vi "TopicRequest_Reply.vi"(2 "Subscriber":T1) -> (0 "XML":string)   [LabVIEW 2012]
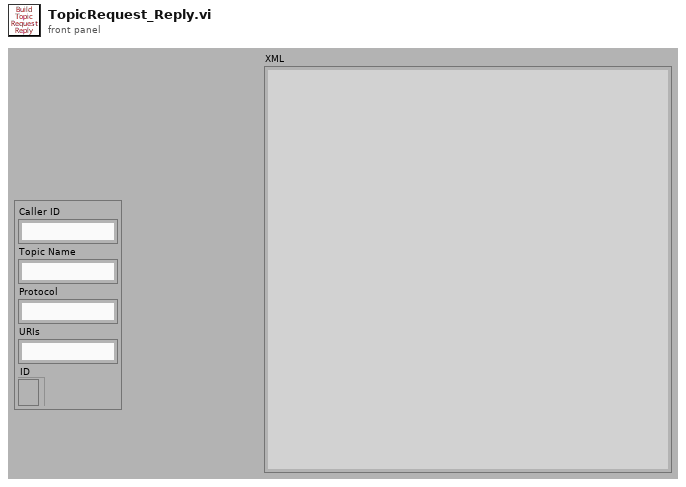
[diagram p1: front panel]
types:
  T1 = cluster{"Caller ID":string, "Topic Name":string, "Protocol":string, "URIs":string, "ID":refnum<k5>}
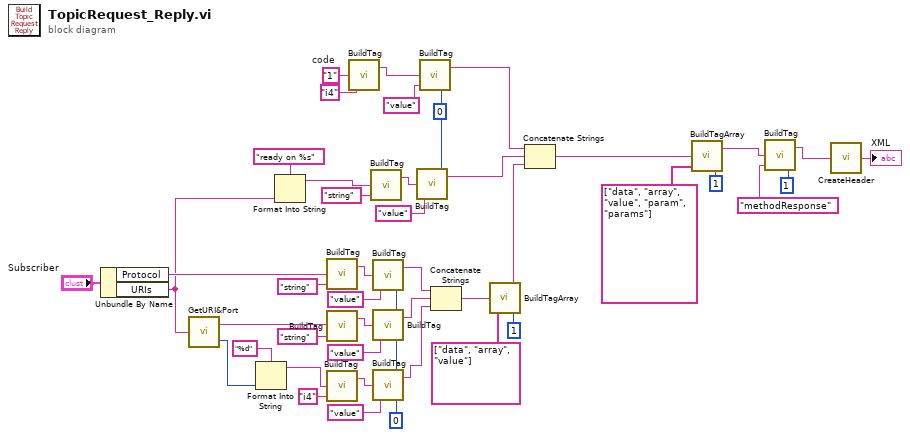
[diagram p0: block diagram]
diagram:
  w12 = i8 0 ("Indent")
  w17 = i8 0 ("Indent")
  w44 = "1"  # code
  n1 = Unbundle By Name("Subscriber") -> ("Protocol"=w28:string, "URIs"=w1:string)
  n2 = call <userlib>:"GetURI&Port.vi"("URI in"=w1) -> ("Port"=w2:u16, "URI"=w3:string)
  n3 = Format Into String(format string="%d", w2) -> (resulting string=w19:string)  [unwired: 2 in, 1 out]
  n4 = Format Into String(format string="ready on %s", w1) -> (resulting string=w39:string)  [unwired: 2 in, 1 out]
  n5 = call <userlib>:"BuildTag.vi"("tag"="string", "value"=w28) -> ("string out"=w31:string)  [unwired: 2 in]
  n6 = call <userlib>:"BuildTag.vi"("tag"="string", "value"=w3) -> ("string out"=w26:string)  [unwired: 2 in]
  n7 = call <userlib>:"BuildTag.vi"("tag"="i4", "value"=w19) -> ("string out"=w21:string)  [unwired: 2 in]
  n8 = call <userlib>:"BuildTag.vi"("tag"="i4", "value"=w44) -> ("string out"=w42:string)  [unwired: 2 in]
  n9 = call <userlib>:"BuildTag.vi"("tag"="string", "value"=w39) -> ("string out"=w37:string)  [unwired: 2 in]
  n10 = call <userlib>:"BuildTag.vi"("Indent"=w17, "tag"="value", "value"=w31) -> ("string out"=w24:string)  [unwired: 1 in]
  n11 = call <userlib>:"BuildTag.vi"("Indent"=w17, "tag"="value", "value"=w26) -> ("string out"=w23:string)  [unwired: 1 in]
  n12 = call <userlib>:"BuildTag.vi"("Indent"=w17, "tag"="value", "value"=w21) -> ("string out"=w18:string)  [unwired: 1 in]
  n13 = call <userlib>:"BuildTag.vi"("Indent"=w12, "tag"="value", "value"=w37) -> ("string out"=w34:string)  [unwired: 1 in]
  n14 = call <userlib>:"BuildTag.vi"("Indent"=w12, "tag"="value", "value"=w42) -> ("string out"=w35:string)  [unwired: 1 in]
  n15 = Concatenate Strings(w24, w23, w18) -> (w16:string)
  n16 = call <userlib>:"BuildTagArray.vi"("Indent"=i8 1, "tags"=string[] ["data", "array", "value"], "value"=w16) -> ("string out"=w13:string)  [unwired: 1 in]
  n17 = Concatenate Strings(w35, w34, w13) -> (w11:string)
  n18 = call <userlib>:"BuildTagArray.vi"("Indent"=i8 1, "tags"=string[] ["data", "array", "value", "param", "params"], "value"=w11) -> ("string out"=w8:string)  [unwired: 1 in]
  n19 = call <userlib>:"BuildTag.vi"("Indent"=i8 1, "tag"="methodResponse", "value"=w8) -> ("string out"=w6:string)  [unwired: 1 in]
  n20 = call <userlib>:"CreateHeader.vi"("Content"=w6) -> ("XML"=→"XML":string)
